vi "ConvertLabviewParameterToMatlabParamData.vi"(8 "BaseName":string, 9 "IgnoreContainerName":bool, 11 "Value":variant) -> (3 "Matlab Param Data":T1[](array[typedef]))   [LabVIEW 2017]
uses:
  Types/MatlabDataBundle.ctl
  Types/MatlabDataType.ctl
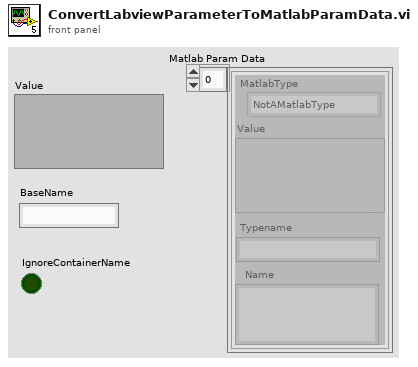
[diagram p1: front panel]
types:
  T1 = typedef "MatlabDataBundle.ctl" = cluster{"MatlabType":T2, "Value":variant, "Name":string, "Typename":string}
  T2 = typedef "MatlabDataType.ctl" = enum16{"NotAMatlabType", "Real", "Complex", "String", "Boolean"}
  T3 = typedef "NI_Data Type.lvlib/Data Type.ctl" = enum8{"Invalid Type", "Void", "I8", "I16", "I32", "I64", "U8", "U16", "U32", "U64", "Single Float", "Double Float", "Extended Float", "Single Complex", "Double Complex", "Extended Complex", "Enum U8", "Enum U16", "Enum U32", "Enum U64", "Single Float With Unit", "Double Float With Unit", "Extended Float With Unit", "Single Complex with Unit", "Double Complex with Unit", "Extended Complex with Unit", "Boolean", "String", "Path", "Picture", "Tag", "Array", "Cluster", "Variant", "LV Variant", "Waveform", "Timestamp", "Digital Waveform", "Digital Data", "ExpressData", "Refnum", "External Data", "VI", "Poly VI", "LabVIEW Class Instance", "Fixed Point"}
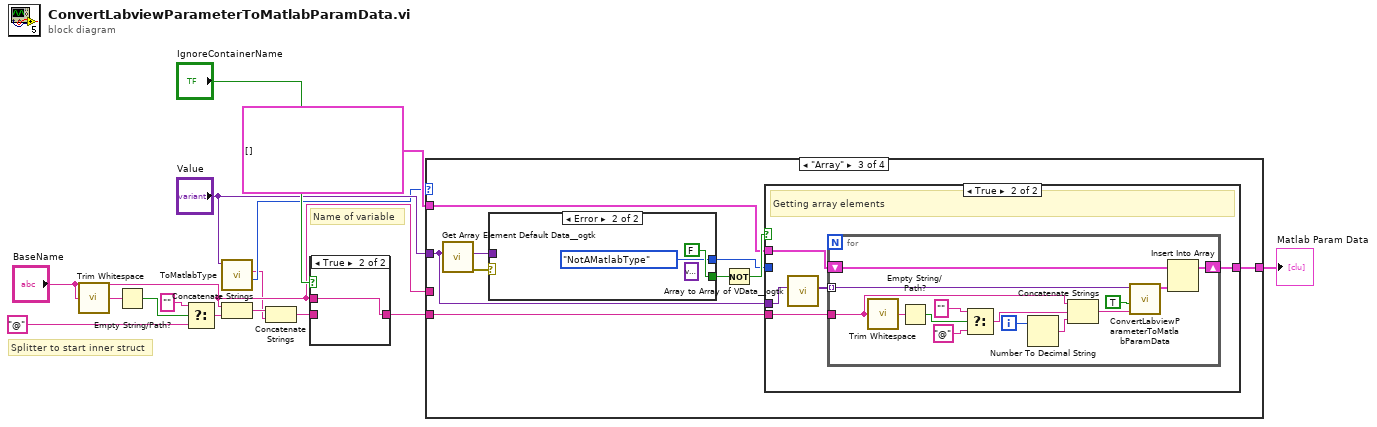
[diagram p0: block diagram]
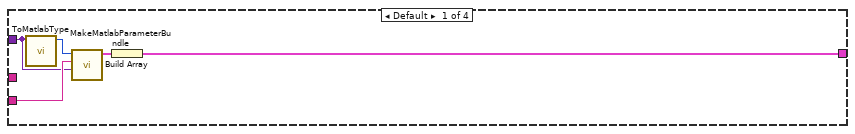
[diagram p3: hidden frame]
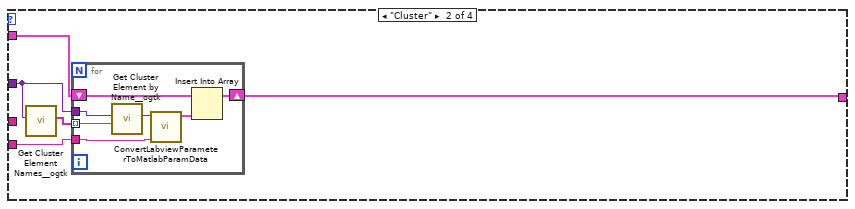
[diagram p4: hidden frame]
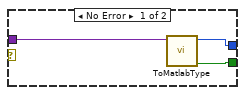
[diagram p5: hidden frame]
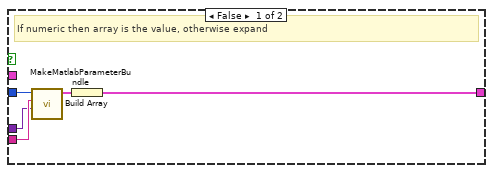
[diagram p6: hidden frame]
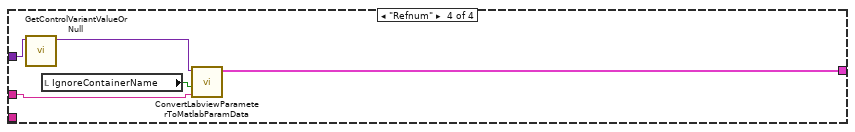
[diagram p7: hidden frame]
diagram:
  # "Splitter to start inner struct"
  # "Name of variable"
  n1 = call <vilib>:"Trim Whitespace.vi"("string"="BaseName") -> ("trimmed string"=w8:string)  [unwired: 1 in]
  n2 = Empty String/Path?(string/path=w8) -> (empty?=w7:bool)
  n3 = Select(t="" ("name"), s=w7, f="@" ("name")) -> (s? t:f=w15:string)
  n4 = call "ToMatlabType.vi"("Value"="Value") -> ("Type"=w2:T3, "Name"=w1:string)  [unwired: 6 in, 3 out]
  n5 = Concatenate Strings("BaseName", w15) -> (w9:string)
  n6 = Concatenate Strings(w9, w1) -> (w11:string)
  n7 = case shown="True" "IgnoreContainerName" {
    tunnel: [w16 w17] -> w12
    tunnel: w11 -> [w16 _]
    tunnel: "BaseName" -> [_ w17]
    frame False {
    }
    frame True {
    }
  }
  n8 = case shown="\"Array\"" w2 {
    tunnel: [w21 w27 w43 w75] -> w5
    tunnel: w12 -> [w19 w26 w40 _]
    tunnel: "BaseName" -> [_ _ _ w76]
    tunnel: T1[] [] -> [_ w24 w39 _]
    tunnel: "Value" -> [w18 w23 w38 w74]
    frame Default {
      n9 = call "ToMatlabType.vi"("Value"=w18) -> ("MatlabType"=w20:T2)  [unwired: 6 in, 4 out]
      n10 = call "MakeMatlabParameterBundle.vi"("value"=w18, "name"=w19, "MatlabType"=w20) -> ("MatlabDataBundle"=w22:T1)  [unwired: 8 in]
      n11 = Build Array(w22) -> (w21:T1[])
    }
    frame "Cluster" {
      n12 = call <userlib>:"Get Cluster Element Names__ogtk.vi"("Cluster"=w23) -> ("Element Names"=w25:string[])  [unwired: 9 in, 1 out]
      n13 = for {
        shift-right: [w34] -> w27
        shift-left: w24 -> [w30]
        tunnel: w26 -> [w33]
        tunnel: w25 -> [w32] mode=indexing
        tunnel: w23 -> [w28]
        n14 = call <userlib>:"Get Cluster Element by Name__ogtk.vi"("Element Name"=w32, "Cluster"=w28) -> ("VElement"=w31:variant)  [unwired: 7 in, 2 out]
        n15 = call "ConvertLabviewParameterToMatlabParamData.vi"("BaseName"=w33, "Value"=w31) -> ("Matlab Param Data"=w29:T1[])  [unwired: 9 in]
        n16 = Insert Into Array(array=w30, new element=w29) -> (w34:T1[])  [unwired: 1 in]
      }
    }
    frame "Array" {
      n17 = call <userlib>:"Get Array Element Default Data__ogtk.vi"("Array"=w38) -> ("error out"=w37:errorcluster, "Array Element Default Data"=w35:variant)  [unwired: 9 in]
      n18 = case shown="Error" w37 {
        tunnel: [w46 FALSE ("IsNumeric")] -> w42
        tunnel: [w45 MatlabDataType."NotAMatlabType" ("MatlabType")] -> w36
        tunnel: w35 -> [w44 _]
        frame No Error {
          n19 = call "ToMatlabType.vi"("Value"=w44) -> ("IsNumeric"=w46:bool, "MatlabType"=w45:T2)  [unwired: 6 in, 3 out]
        }
        frame Error {
          (unwired) variant
        }
      }
      n20 = Not(x=w42) -> (.not. x?=w41:bool)
      n21 = case shown="True" w41 {
        tunnel: [w51 w58] -> w43
        tunnel: w40 -> [w53 w57]
        tunnel: w39 -> [_ w56]
        tunnel: w38 -> [w50 w55]
        tunnel: w36 -> [w49 _]
        frame False {
          # "If numeric then array is the value, otherwise expand"
          n22 = call "MakeMatlabParameterBundle.vi"("value"=w50, "name"=w53, "MatlabType"=w49) -> ("MatlabDataBundle"=w52:T1)  [unwired: 8 in]
          n23 = Build Array(w52) -> (w51:T1[])
        }
        frame True {
          # "Getting array elements"
          n24 = call <userlib>:"Array to Array of VData__ogtk.vi"("MultiD Array"=w55) -> ("1D Array of Variants"=w54:variant[])  [unwired: 9 in, 1 out]
          n25 = for {
            shift-right: [w72] -> w58
            shift-left: w56 -> [w68]
            tunnel: w57 -> [w63]
            tunnel: w54 -> [w65] mode=indexing
            i -> [w66]
            n26 = call <vilib>:"Trim Whitespace.vi"("string"=w63) -> ("trimmed string"=w64:string)  [unwired: 1 in]
            n27 = Empty String/Path?(string/path=w64) -> (empty?=w62:bool)
            n28 = Select(t="", s=w62, f="@" ("string")) -> (s? t:f=w59:string)
            n29 = Number To Decimal String(number=w66) -> (decimal integer string=w71:string)  [unwired: 1 in]
            n30 = Concatenate Strings(w63, w59, w71) -> (w70:string)
            n31 = call "ConvertLabviewParameterToMatlabParamData.vi"("BaseName"=w70, "IgnoreContainerName"=TRUE, "Value"=w65) -> ("Matlab Param Data"=w67:T1[])  [unwired: 8 in]
            n32 = Insert Into Array(array=w68, new element=w67) -> (w72:T1[])  [unwired: 1 in]
          }
        }
      }
    }
    frame "Refnum" {
      n33 = call "GetControlVariantValueOrNull.vi"("ControlVariant"=w74) -> ("Value"=w77:variant)  [unwired: 9 in, 1 out]
      n34 = local read "IgnoreContainerName"() -> (w73:bool)
      n35 = call "ConvertLabviewParameterToMatlabParamData.vi"("BaseName"=w76, "IgnoreContainerName"=w73, "Value"=w77) -> ("Matlab Param Data"=w75:T1[])  [unwired: 8 in]
    }
  }
  "Matlab Param Data" <- w5
